vi "Single Encoder Data.vi"(9 "Tick Constant":dbl, 10 "Rate":dbl, 11 "Distance":dbl) -> (2 "output cluster":T1)   [LabVIEW 2015]
uses:
  Common Code/Encoder Values.ctl
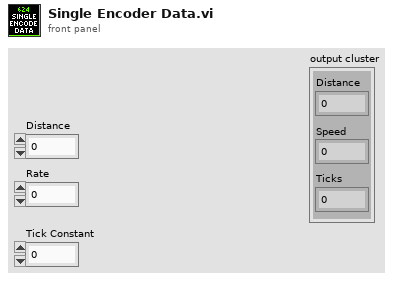
[diagram p1: front panel]
types:
  T1 = typedef "Encoder Values.ctl" = cluster{"Distance":dbl, "Speed":dbl, "Ticks":dbl}
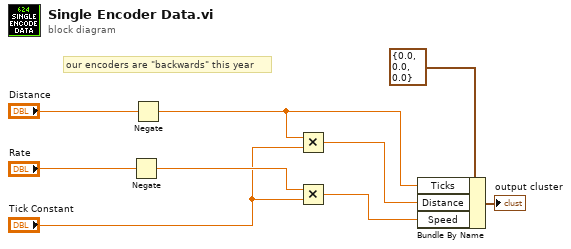
[diagram p0: block diagram]
diagram:
  # "our encoders are \"backwards\" this year"
  n1 = Negate(x="Rate") -> (-x=w4:dbl)
  n2 = Negate(x="Distance") -> (-x=w6:dbl)
  n3 = Multiply(x=w6, y="Tick Constant") -> (x*y=w9:dbl)
  n4 = Multiply(x=w4, y="Tick Constant") -> (x*y=w8:dbl)
  n5 = Bundle By Name(cluster=T1 {"Distance"=0.0, "Speed"=0.0, "Ticks"=0.0} ("Encoder Values"), "Ticks"=w6, "Distance"=w9, "Speed"=w8) -> (→"output cluster":T1)
